vi "UpdateNode.vi"(8 "Cost":dbl, 9 "y":i32, 10 "x":i32, 11 "OccupancyGridWorldMap in":refnum<class "NI_Robotics_OccupancyGridWorldMap.lvclass">) -> (3 "OccupancyGridWorldMap out":refnum<class "NI_Robotics_OccupancyGridWorldMap.lvclass">)   [LabVIEW 2017, in "NI_Robotics_OccupancyGridWorldMap.lvclass"]
uses:
  <vilib>/robotics/Navigation/shared/WorldMap/OccupancyGridWorldMap/NI_Robotics_OccupancyGridWorldMap.lvclass
  <vilib>/robotics/Navigation/shared/WorldMap/OccupancyGridWorldMap/NI_Robotics_OccupancyGridWorldMap.lvclass/NI_Robotics_OccupancyGridWorldMap.ctl
  <vilib>/robotics/Navigation/shared/MapNode/OccupancyGridNode/NI_Robotics_OccupancyGridMapNode.lvclass
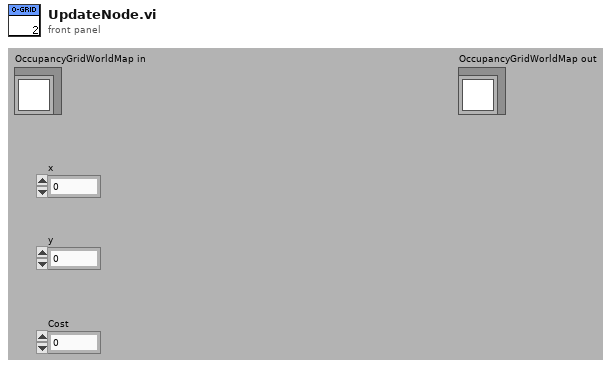
[diagram p1: front panel]
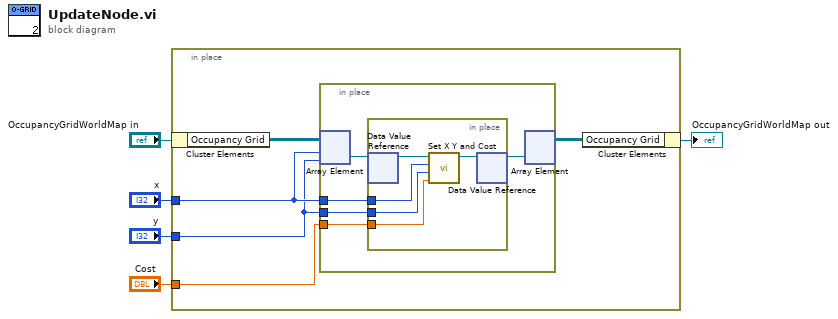
[diagram p0: block diagram]
diagram:
  n1 = in-place {
    in-place-border: "x" -> [w7]
    in-place-border: "y" -> [w6]
    in-place-border: "Cost" -> [w8]
    n2 = in-place-cluster #1("OccupancyGridWorldMap in") -> ("Occupancy Grid"=w10:refnum<data-value>[][])
    n3 = in-place {
      in-place-border: w8 -> [w13]
      in-place-border: w7 -> [w12]
      in-place-border: w6 -> [w11]
      n4 = in-place-array #2(w10, w7, w6) -> (w15:refnum<data-value>)
      n5 = in-place {
        in-place-border: w13 -> [w20]
        in-place-border: w12 -> [w17]
        in-place-border: w11 -> [w16]
        n6 = in-place-dvr #3(w15) -> (w19:refnum<class "NI_Robotics_OccupancyGridMapNode.lvclass">)  [unwired: 1 out]
        n7 = call-dynamic "Set X Y and Cost.vi"("Cost"=w20, "y"=w16, "x"=w17, "OccupancyGridMapNode in"=w19) -> ("OccupancyGridMapNode out"=w18:refnum<class "NI_Robotics_OccupancyGridMapNode.lvclass">)  [unwired: 7 in]
        n8 = in-place-dvr #3(w18) -> (w14:refnum<data-value>)  [unwired: 1 out]
      }
      n9 = in-place-array #2(w14) -> (w9:refnum<data-value>[][])  [unwired: 2 out]
    }
    n10 = in-place-cluster #1("Occupancy Grid"=w9) -> (→"OccupancyGridWorldMap out":refnum<class "NI_Robotics_OccupancyGridWorldMap.lvclass">)
  }
